vi "Items.vi"(11 "JSONMessage in":refnum<class "WampMessage JSON.lvclass">) -> (2 "<JSON>Elements":string[](array[string]), 3 "JSONMessage out":refnum<class "WampMessage JSON.lvclass">)   [LabVIEW 2020, in "wamplv.lvlib" / "WampMessage JSON.lvclass"]
uses:
  WampMessage JSON.lvclass
  WampMessage JSON.lvclass/WampMessage JSON.ctl
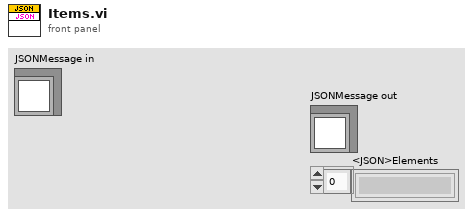
[diagram p1: front panel]
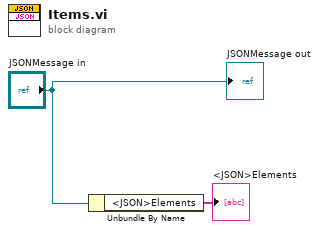
[diagram p0: block diagram]
diagram:
  n1 = Unbundle By Name("JSONMessage in") -> ("<JSON>Elements"=→"<JSON>Elements":string[])
  "JSONMessage out" <- "JSONMessage in"
